vi "test_libssh2_channel_setenv_ex.vi"() -> ()   [LabVIEW 2017, in "integration_tests.lvlib"]
uses:
  integration_tests.lvlib
  libssh2/libssh2_channel_open_ex.vi
  libssh2/libssh2_channel_process_startup.vi
  libssh2/libssh2_channel_read_ex.vi
  support/support.lvlib
  libssh2/libssh2.lvlib
  <vilib>/PNR/Transparent Assertions/Transparent Assertions/Transparent Assertions.lvlib
panel:
  out "error out":errorcluster
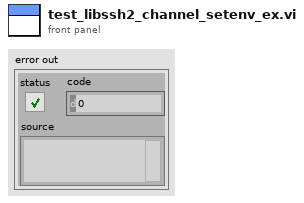
[diagram p1: front panel]
types:
  T1 = typedef "libssh2.lvlib/Session Refnum.ctl" = refnum<k1>
  T2 = typedef "libssh2.lvlib/Channel Refnum.ctl" = refnum<k1>
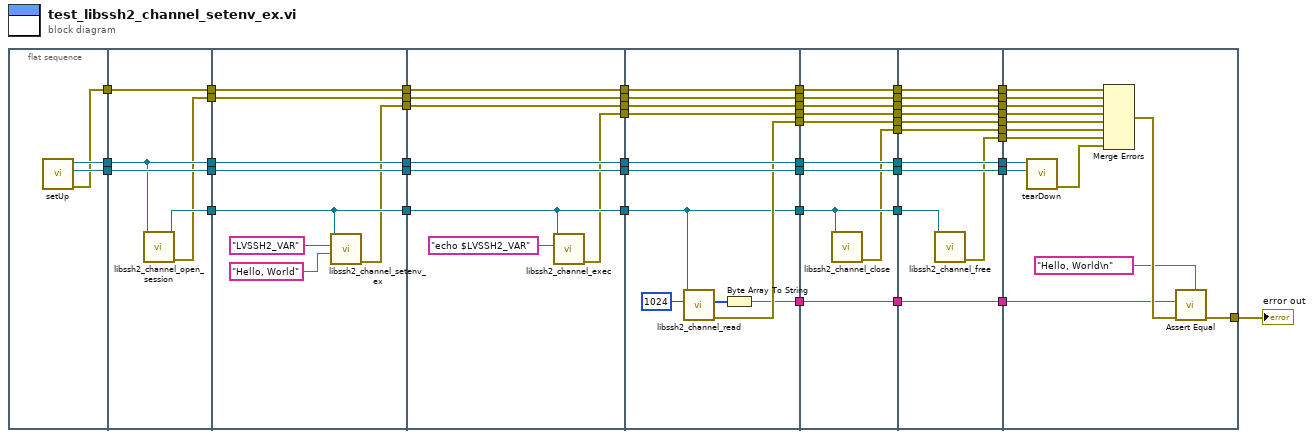
[diagram p0: block diagram]
diagram:
  n1 = flat-sequence {
    tunnel: [w54] -> w51
    tunnel: [w53] -> w50
    tunnel: [w52] -> w49
    tunnel: w51 -> [w58]
    tunnel: w50 -> [w59]
    tunnel: [w58] -> w48
    tunnel: [w59] -> w47
    tunnel: [w57] -> w46
    tunnel: w49 -> [w56]
    tunnel: [w56] -> w45
    tunnel: [w55] -> w44
    tunnel: w48 -> [w67]
    tunnel: [w67] -> w17
    tunnel: w47 -> [w66]
    tunnel: [w66] -> w15
    tunnel: w46 -> [w62]
    tunnel: [w62] -> w13
    tunnel: w45 -> [w65]
    tunnel: [w65] -> w11
    tunnel: w44 -> [w64]
    tunnel: [w64] -> w9
    tunnel: [w61] -> w7
    tunnel: w17 -> [w75]
    tunnel: [w75] -> w16
    tunnel: w15 -> [w74]
    tunnel: [w74] -> w14
    tunnel: w13 -> [w70]
    tunnel: [w70] -> w12
    tunnel: w11 -> [w73]
    tunnel: [w73] -> w10
    tunnel: w9 -> [w72]
    tunnel: [w72] -> w8
    tunnel: w7 -> [w71]
    tunnel: [w71] -> w6
    tunnel: [w68] -> w5
    tunnel: w16 -> [w86]
    tunnel: [w86] -> w43
    tunnel: w14 -> [w85]
    tunnel: [w85] -> w42
    tunnel: w12 -> [w76]
    tunnel: [w76] -> w41
    tunnel: w10 -> [w84]
    tunnel: [w84] -> w40
    tunnel: w8 -> [w83]
    tunnel: [w83] -> w39
    tunnel: w6 -> [w82]
    tunnel: [w82] -> w38
    tunnel: [w79] -> w37
    tunnel: [w77] -> w36
    tunnel: w5 -> [w81]
    tunnel: [w81] -> w4
    tunnel: w43 -> [w96]
    tunnel: w42 -> [w95]
    tunnel: w41 -> [w94]
    tunnel: [w96] -> w35
    tunnel: [w95] -> w34
    tunnel: [w88] -> w33
    tunnel: [w94] -> w32
    tunnel: [w93] -> w31
    tunnel: w40 -> [w92]
    tunnel: [w92] -> w30
    tunnel: w39 -> [w91]
    tunnel: [w91] -> w29
    tunnel: w38 -> [w90]
    tunnel: [w90] -> w28
    tunnel: w37 -> [w89]
    tunnel: [w89] -> w27
    tunnel: w36 -> [w88]
    tunnel: w4 -> [w87]
    tunnel: [w87] -> w3
    tunnel: w35 -> [w107]
    tunnel: w34 -> [w106]
    tunnel: w33 -> [w105]
    tunnel: w32 -> [w104]
    tunnel: [w107] -> w26
    tunnel: [w106] -> w25
    tunnel: [w105] -> w24
    tunnel: [w103] -> w23
    tunnel: w31 -> [w102]
    tunnel: [w102] -> w22
    tunnel: w30 -> [w101]
    tunnel: [w101] -> w21
    tunnel: w29 -> [w100]
    tunnel: [w100] -> w20
    tunnel: w28 -> [w99]
    tunnel: [w99] -> w19
    tunnel: w27 -> [w98]
    tunnel: [w98] -> w18
    tunnel: w3 -> [w97]
    tunnel: [w97] -> w2
    tunnel: w26 -> [w121]
    tunnel: w25 -> [w120]
    tunnel: w24 -> [w110]
    tunnel: [w119] -> w1
    tunnel: w23 -> [w117]
    tunnel: w22 -> [w116]
    tunnel: w21 -> [w115]
    tunnel: w20 -> [w113]
    tunnel: w19 -> [w112]
    tunnel: w18 -> [w111]
    tunnel: w2 -> [w109]
    frame #0 {
      n2 = call "setUp.vi"() -> ("error out"=w52:errorcluster, "connection ID"=w53:refnum<k5>, "session"=w54:T1)  [unwired: 9 in]
    }
    frame #1 {
      n3 = call "libssh2_channel_open_session.vi"("session"=w58) -> ("error out"=w55:errorcluster, "channel"=w57:T2)  [unwired: 9 in]
    }
    frame #2 {
      n4 = call "libssh2_channel_setenv_ex.vi"("value"="Hello, World", "varname"="LVSSH2_VAR", "channel"=w62) -> ("error out"=w61:errorcluster)  [unwired: 8 in]
    }
    frame #3 {
      n5 = call "libssh2_channel_exec.vi"("command"="echo $LVSSH2_VAR", "channel"=w70) -> ("error out"=w68:errorcluster)  [unwired: 9 in]
    }
    frame #4 {
      n6 = call "libssh2_channel_read.vi"("buffer length"=1024, "channel"=w76) -> ("error out"=w79:errorcluster, "buffer"=w78:u8[])  [unwired: 8 in]
      n7 = Byte Array To String(unsigned byte array=w78) -> (string=w77:string)
    }
    frame #5 {
      n8 = call "libssh2_channel_close.vi"("channel"=w94) -> ("error out"=w93:errorcluster)  [unwired: 10 in]
    }
    frame #6 {
      n9 = call "libssh2_channel_free.vi"("channel"=w104) -> ("error out"=w103:errorcluster)  [unwired: 10 in]
    }
    frame #7 {
      n10 = call "tearDown.vi"("connection ID"=w120, "session"=w121) -> ("error out"=w118:errorcluster)  [unwired: 9 in]
      n11 = Merge Errors(w115, w113, w112, w109, w111, w116, w117, w118) -> (w114:errorcluster)
      n12 = call <vilib>:"Assert Equal.vi"("Expected"="Hello, World\n" ("value"), "error in (no error)"=w114, "Actual"=w110) -> ("error out"=w119:errorcluster)  [unwired: 8 in]
    }
  }
  "error out" <- w1
